vi "Byte Buffer.Read (Boolean).vi"(8 "error in (no error)":errorcluster, 10 "buffer offset":u64, 11 "Byte Buffer in":refnum<class "Byte Buffer.lvclass">) -> (0 "error out":errorcluster, 1 "value":bool, 3 "Byte Buffer out":refnum<class "Byte Buffer.lvclass">)   [LabVIEW 2016, in "VeriStand Data.lvlib" / "Byte Buffer.lvclass"]
doc: "Reads one element of data from the provided <B>Byte Buffer</B> at location <B>buffer offset</B> in the format of the data type specified."
uses:
  Byte Buffer.lvclass
  Byte Buffer.lvclass/Byte Buffer.ctl
  Byte Buffer.Read (String).vi
  Byte Buffer.Allocate.vi
  Byte Buffer.Buffer Subset.Get.vi
  Memory Management/Memory Management.MoveByteBlock.Write (String).vi
  Memory Management/Memory Management.Handle Return.vi
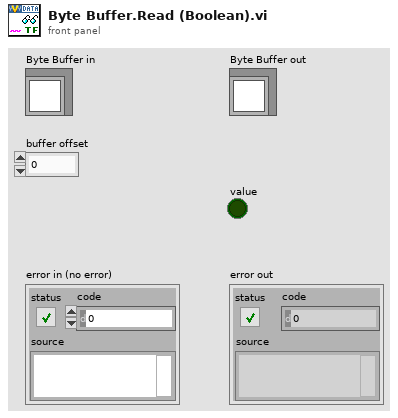
[diagram p1: front panel]
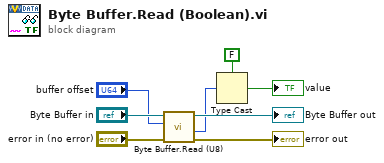
[diagram p0: block diagram]
diagram:
  n1 = call "Byte Buffer.Read (U8).vi"("error in (no error)"="error in (no error)", "buffer offset"="buffer offset", "Byte Buffer in"="Byte Buffer in") -> ("error out"=→"error out":errorcluster, "value"=w3:u8, "Byte Buffer out"=→"Byte Buffer out":refnum<class "Byte Buffer.lvclass">)  [unwired: 6 in]
  n2 = Type Cast(type=FALSE, x=w3) -> (*(type *) &x=→"value":bool)
